vi "MDAQ_READ_Spectrum.vi"(8 "error in":errorcluster, 9 "Status_Cluster IN":T1 {"GATESTOP" format="%04x"; "GATESTRT" format="%04x"; "AMPLITUDE" format="%04x"; "M_CYCLES" format="%04x"; "N_CYCLES" format="%04x"; "STEP" format="%04x"; "BASE" format="%04x"; "CHAN" format="%04x"}, 10 "Mode":enum16{"BIN", "ASCII"}(ring), 11 "VISA resource name":refnum<visa-resource-name>) -> (0 "error out":errorcluster, 1 "output cluster":T1 {"GATESTOP" format="%04x"; "GATESTRT" format="%04x"; "AMPLITUDE" format="%04x"; "M_CYCLES" format="%04x"; "N_CYCLES" format="%04x"; "STEP" format="%04x"; "BASE" format="%04x"; "CHAN" format="%04x"}, 2 "Output Array":u32[](array[numeric]), 3 "VISA resource name out":refnum<visa-resource-name>)   [LabVIEW 2021]
uses:
  Status_Cluster.ctl
  dfacd9d0-e592-4c9f-9d6b-37ae124cbe0a.vi
  1ff17288-4105-4d09-adc0-fb781dd7377f.vi
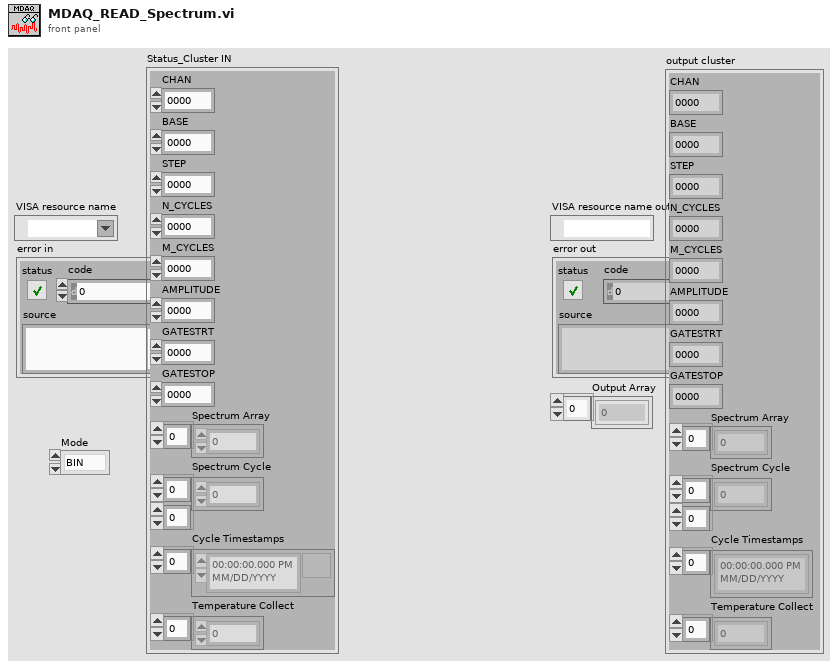
[diagram p1: front panel]
types:
  T1 = typedef "Status_Cluster.ctl" = cluster{"CHAN":u32, "BASE":u32, "STEP":u32, "N_CYCLES":u32, "M_CYCLES":u32, "AMPLITUDE":u32, "GATESTRT":u32, "GATESTOP":u32, "Spectrum Array":u32[], "Spectrum Cycle":u32[][], "Cycle Timestamps":timestamp[], "Temperature Collect":dbl[]}
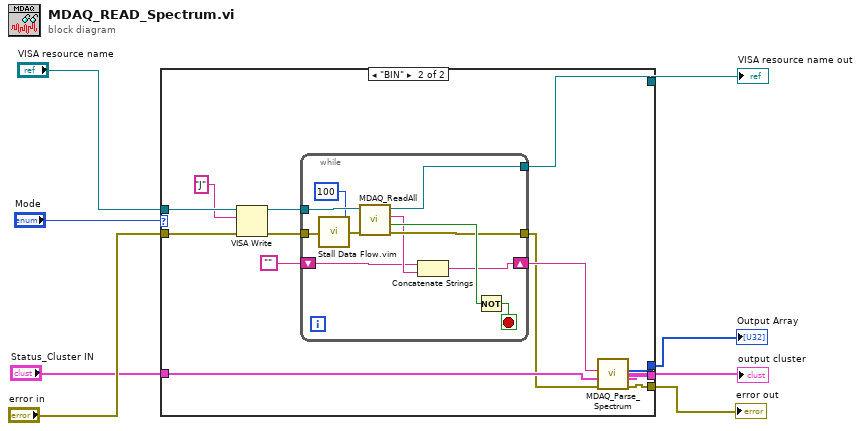
[diagram p0: block diagram]
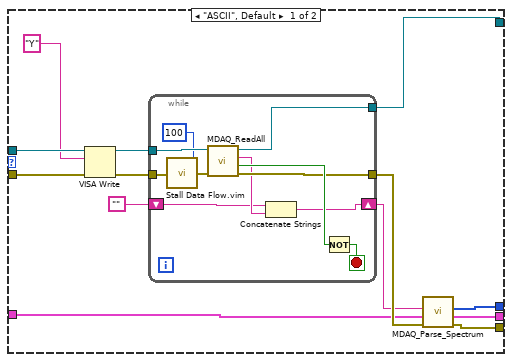
[diagram p2: hidden frame]
diagram:
  n1 = case shown="\"BIN\"" "Mode" {
    tunnel: "VISA resource name" -> [w21 w45]
    tunnel: "error in" -> [w20 w44]
    tunnel: [w18 w42] -> w6
    tunnel: "Status_Cluster IN" -> [w13 w34]
    tunnel: [w11 w36] -> w3
    tunnel: [w10 w37] -> w2
    tunnel: [w9 w38] -> w1
    frame "ASCII", Default {
      n2 = VISA Write(VISA resource name=w21, write buffer="Y", error in (no error)=w20) -> (VISA resource name out=w19:refnum<visa-resource-name>, error out=w16:errorcluster)  [unwired: 1 out]
      n3 = while {
        tunnel: w19 -> [w32]
        tunnel: [w31] -> w18
        tunnel: [w28] -> w14
        shift-right: [w25] -> w12
        shift-left: "" -> [w26]
        tunnel: w16 -> [w24]
        stop <- w30 stop-if-true
        n4 = call "Stall Data Flow.vim"("value in"=w24, "milliseconds to wait"=u32 100) -> ("value out"=w23:errorcluster)  [unwired: 1 out]
        n5 = call "MDAQ_ReadAll.vi"("error in"=w23, "VISA resource name"=w32) -> ("error IO"=w28:errorcluster, "Buffer Not Empty"=w29:bool, "read buffer"=w27:string, "VISA resource name out"=w31:refnum<visa-resource-name>)  [unwired: 6 in]
        n6 = Concatenate Strings(w26, w27) -> (w25:string)
        n7 = Not(x=w29) -> (.not. x?=w30:bool)
      }
      n8 = call "MDAQ_Parse_Spectrum.vi"("error in"=w14, 9:w13, "input buffer"=w12) -> ("error out"=w11:errorcluster, "output cluster"=w10:T1, "Array"=w9:u32[])  [unwired: 6 in]
    }
    frame "BIN" {
      n9 = VISA Write(VISA resource name=w45, write buffer="J", error in (no error)=w44) -> (VISA resource name out=w43:refnum<visa-resource-name>, error out=w40:errorcluster)  [unwired: 1 out]
      n10 = while {
        tunnel: w43 -> [w56]
        tunnel: [w55] -> w42
        tunnel: [w52] -> w33
        shift-right: [w49] -> w35
        shift-left: "" -> [w50]
        tunnel: w40 -> [w48]
        stop <- w54 stop-if-true
        n11 = call "Stall Data Flow.vim"("value in"=w48, "milliseconds to wait"=u32 100) -> ("value out"=w47:errorcluster)  [unwired: 1 out]
        n12 = call "MDAQ_ReadAll.vi"("error in"=w47, "VISA resource name"=w56) -> ("error IO"=w52:errorcluster, "Buffer Not Empty"=w53:bool, "read buffer"=w51:string, "VISA resource name out"=w55:refnum<visa-resource-name>)  [unwired: 6 in]
        n13 = Concatenate Strings(w50, w51) -> (w49:string)
        n14 = Not(x=w53) -> (.not. x?=w54:bool)
      }
      n15 = call "MDAQ_Parse_Spectrum.vi"("error in"=w33, 9:w34, "input buffer"=w35) -> ("error out"=w36:errorcluster, "output cluster"=w37:T1, "Array"=w38:u32[])  [unwired: 6 in]
    }
  }
  "VISA resource name out" <- w6
  "error out" <- w3
  "output cluster" <- w2
  "Output Array" <- w1
